vi "HV Verify PMT Settings.vi"(8 "PMT's":string[](array[string]), 11 "Test":string) -> (3 "Voltages":string[](array[string]))   [LabVIEW 2018, in "HV QMH.lvlib"]
uses:
  HV QMH.lvlib
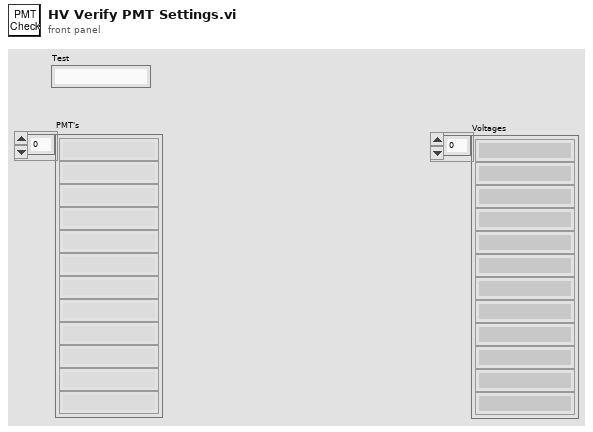
[diagram p1: front panel]
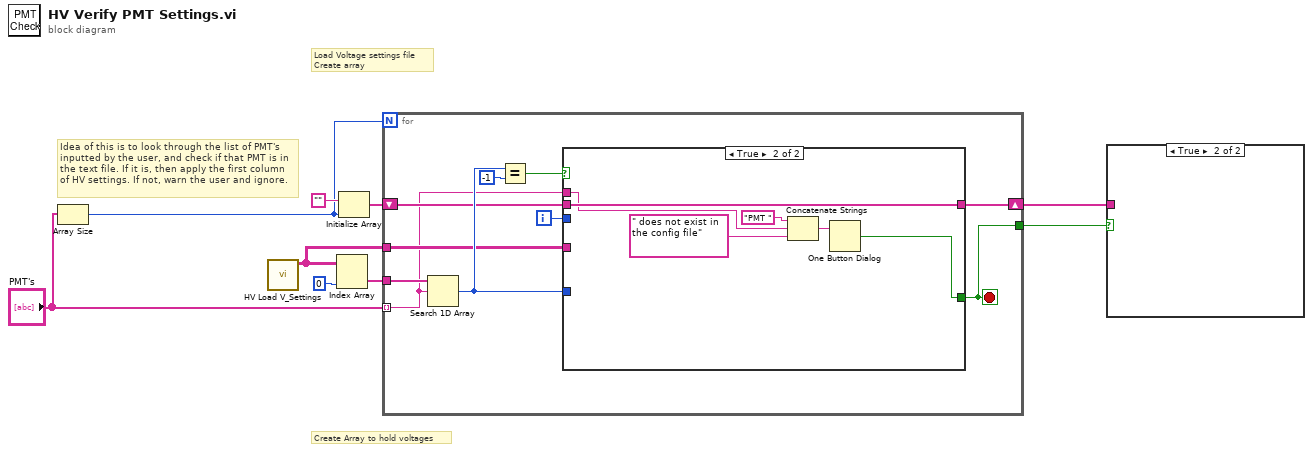
[diagram p0: block diagram]
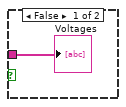
[diagram p2: hidden frame]
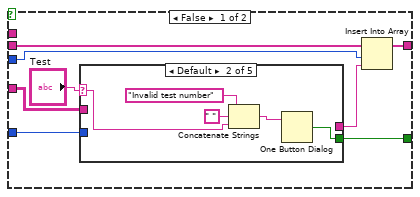
[diagram p3: hidden frame]
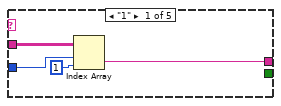
[diagram p4: hidden frame]
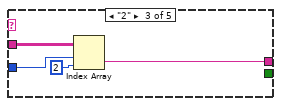
[diagram p5: hidden frame]
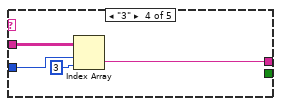
[diagram p6: hidden frame]
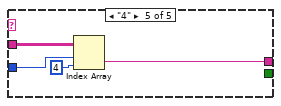
[diagram p7: hidden frame]
diagram:
  # "Load Voltage settings file\nCreate array"
  # "Create Array to hold voltages"
  # "Idea of this is to look through the list of PMT's inputted by the user, and check if that PMT is in the text file. If it is, then apply the first column of HV settings. If not, warn the user and ignore."
  n1 = Array Size(array="PMT's") -> (size(s)=w2:i32)
  n2 = call "HV Load V_Settings.vi"() -> ("V_Settings"=w3:string[][])  [unwired: 9 in, 2 out]
  n3 = Index Array(array=w3, index (col)=0) -> (element=w4:string[])  [unwired: 1 in]
  n4 = Initialize Array("", w2) -> (w7:string[])
  n5 = for {
    N: w2 -> [_]
    tunnel: "PMT's" -> [w11] mode=indexing
    shift-right: [w12] -> w6
    shift-left: w7 -> [w14]
    tunnel: w4 -> [w15]
    tunnel: w3 -> [w16]
    tunnel: [w10] -> w1
    i -> [w13]
    stop <- w10 stop-if-true
    n6 = Search 1D Array(1D array=w15, element=w11) -> (index of element=w17:i32)  [unwired: 1 in]
    n7 = Equal?(x=w17, y=-1) -> (x = y?=w19:bool)
    n8 = case shown="True" w19 {
      tunnel: w17 -> [w26 _]
      tunnel: w16 -> [w27 _]
      tunnel: w14 -> [w25 w54]
      tunnel: w13 -> [w24 _]
      tunnel: [w22 w54] -> w12
      tunnel: w11 -> [_ w52]
      tunnel: [w20 w49] -> w10
      frame False {
        n9 = case shown="Default" "Test" {
          selector: "Test" -> [_ w32 _ _ _]
          tunnel: w27 -> [w31 _ w40 w44 w48]
          tunnel: w26 -> [w30 _ w39 w43 w47]
          tunnel: [w28 _ w37 w41 w45] -> w23
          tunnel: [_ w36 _ _ _] -> w20
          frame "1" {
            n10 = Index Array(array=w31, index (row)=w30, index (col)=1) -> (element=w28:string)
          }
          frame Default {
            n11 = Concatenate Strings("Invalid test number" ("message"), " " ("string"), w32) -> (w35:string)
            n12 = One Button Dialog(message=w35) -> (true=w36:bool)  [unwired: 1 in]
          }
          frame "2" {
            n13 = Index Array(array=w40, index (row)=w39, index (col)=2) -> (element=w37:string)
          }
          frame "3" {
            n14 = Index Array(array=w44, index (row)=w43, index (col)=3) -> (element=w41:string)
          }
          frame "4" {
            n15 = Index Array(array=w48, index (row)=w47, index (col)=4) -> (element=w45:string)
          }
        }
        n16 = Insert Into Array(array=w25, index=w24, new element=w23) -> (w22:string[])
      }
      frame True {
        n17 = Concatenate Strings("PMT ", w52, " does not exist in the config file") -> (w50:string)
        n18 = One Button Dialog(message=w50) -> (true=w49:bool)  [unwired: 1 in]
      }
    }
  }
  n19 = case shown="True" w1 {
    tunnel: w6 -> [w55 _]
    frame False {
      "Voltages" <- w55
    }
    frame True {
    }
  }
